vi "Obtain control updates queue.vi"(8 "error in (no error)":errorcluster, 11 "Fiber Auto Collimation panel":refnum<class "Fiber Auto Collimation panel.lvclass">) -> (0 "error out":errorcluster, 3 "Update control(s) queue out":refnum<queue>)   [LabVIEW 2018, in "Fiber Auto Collimation References.lvclass"]
doc: "Gets the reference to the queue for listing which control(s) need to be updated (usually after a state data update). The queue reference is specific to the panel type and clone name of the reference passed in."
uses:
  Fiber Auto Collimation References.lvclass
  Panels/Fiber Auto Collimation panel.lvclass
  C:/Program Files (x86)/National Instruments/LabVIEW 2018/user.lib/nLight Tidbits/Cross-library references/Cross-library key/Cross-library key.lvclass
  bbbe1298-683a-40aa-a8c7-7440d6b00167.vi
  6fc5f598-48c0-4917-9816-ab627c4e60eb.vi
  bbbe1298-683a-40aa-a8c7-7440d6b00167.vi/d76dba9b-d1d7-425e-97b2-ec087d95774d.vi
  <userlib>/nLight Tidbits/Cross-library references/Cross-library key/Obtain cross library semaphore and acquire.vi
  bbbe1298-683a-40aa-a8c7-7440d6b00167.vi/16c40fe3-e9f6-49e5-ae84-44dc056e7d5b.vi
  6fc5f598-48c0-4917-9816-ab627c4e60eb.vi/8a601b95-9472-4233-99ca-0d82ade4dafb.vi
  6fc5f598-48c0-4917-9816-ab627c4e60eb.vi/cb6b160f-814f-40b7-ba5e-cb6ca000a881.vi
  <userlib>/nLight Error Handling/Trash error.vi
  <vilib>/Utility/error.llb/Clear Errors.vi
  <vilib>/Utility/semaphor.llb/Obtain Semaphore Reference.vi
  <vilib>/Utility/semaphor.llb/Acquire Semaphore.vi
  <userlib>/nLight Error Handling/Log any errors.vi
  <userlib>/nLight Tidbits/Cross-library references/Cross-library key/Obtain class key.vi
  <vilib>/Utility/semaphor.llb/Release Semaphore.vi
  <vilib>/Utility/semaphor.llb/Release Semaphore Reference.vi
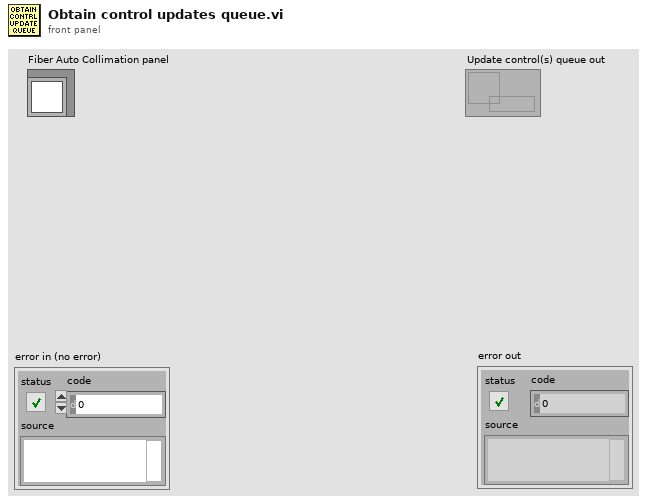
[diagram p1: front panel]
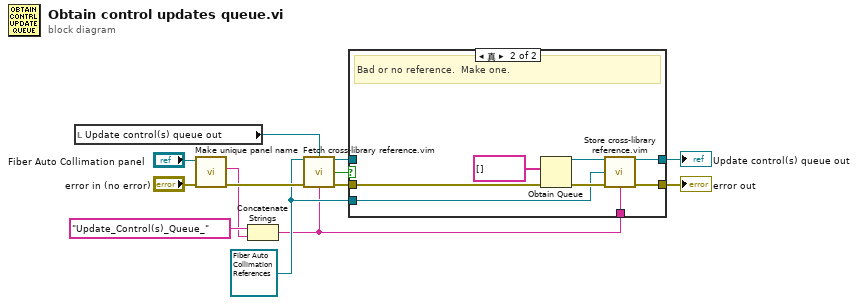
[diagram p0: block diagram]
diagram:
  w7 = refnum<class "Fiber Auto Collimation References.lvclass"> refnum ("nLight Station Template References.lvclass")
  n1 = local read "Update control(s) queue out"() -> (w1:refnum<queue>)
  n2 = call "Make unique panel name.vi"("error in (no error)"="error in (no error)", "Fiber Auto Collimation panel in"="Fiber Auto Collimation panel") -> ("error out"=w9:errorcluster, "Unique panel name"=w3:string)  [unwired: 7 in, 1 out]
  n3 = Concatenate Strings("Update_Control(s)_Queue_", w3) -> (w2:string)
  n4 = call "Fetch cross-library reference.vim"("Cross-library key"=w7, "Reference type to fetch"=w1, "error in (no error)"=w9, "Specific ref type name [String/Enum]"=w2) -> ("Stored value (if present)"=w8:refnum<queue>, "Nothing to fetch OR bad reference"=w5:bool, "error out"=w6:errorcluster)  [unwired: 9 in]
  n5 = case shown="真" w5 {
    tunnel: w6 -> [w14 w23]
    tunnel: [w14 w18] -> w13
    tunnel: [w15 w17] -> w12
    tunnel: w8 -> [w15 _]
    tunnel: w7 -> [_ w20]
    tunnel: w2 -> [_ w19]
    frame False {
      # "Good reference last time.  Pass it out again."
    }
    frame True {
      # "Bad or no reference.  Make one."
      n6 = Obtain Queue(element data type=string[] [], error in (no error)=w23) -> (queue out=w16:refnum<queue>, error out=w21:errorcluster)  [unwired: 3 in, 1 out]
      n7 = call "Store cross-library reference.vim"("Reference to store"=w16, "Cross-library key"=w20, "error in (no error)"=w21, "Specific ref type name [String/Enum]"=w19) -> ("Copy of stored reference"=w17:refnum<queue>, "error out"=w18:errorcluster)  [unwired: 8 in, 2 out]
    }
  }
  "error out" <- w13
  "Update control(s) queue out" <- w12
